vi "GetArmCount.vi"(8 "Error In":errorcluster, 11 "Keithley 7001 In":refnum<visa-resource-name>) -> (0 "Error Out":errorcluster, 1 "Infinite?":bool, 2 "Count?":u32, 3 "Keithley 7001 Out":refnum<visa-resource-name>)   [LabVIEW 2012, in "Keithley-7001.lvlib"]
uses:
  Keithley-7001.lvlib
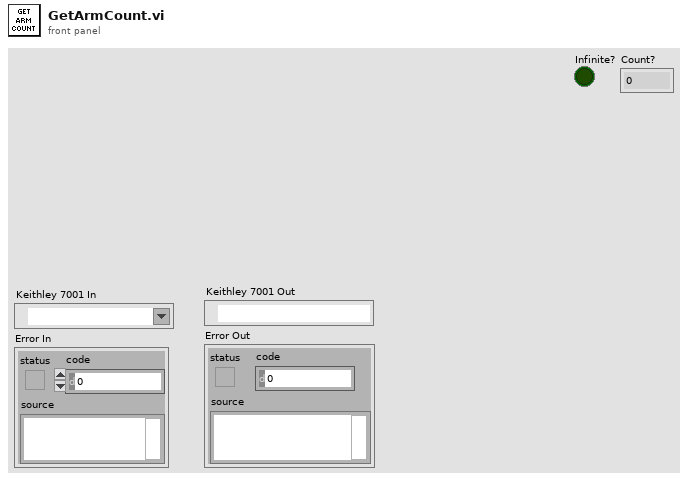
[diagram p1: front panel]
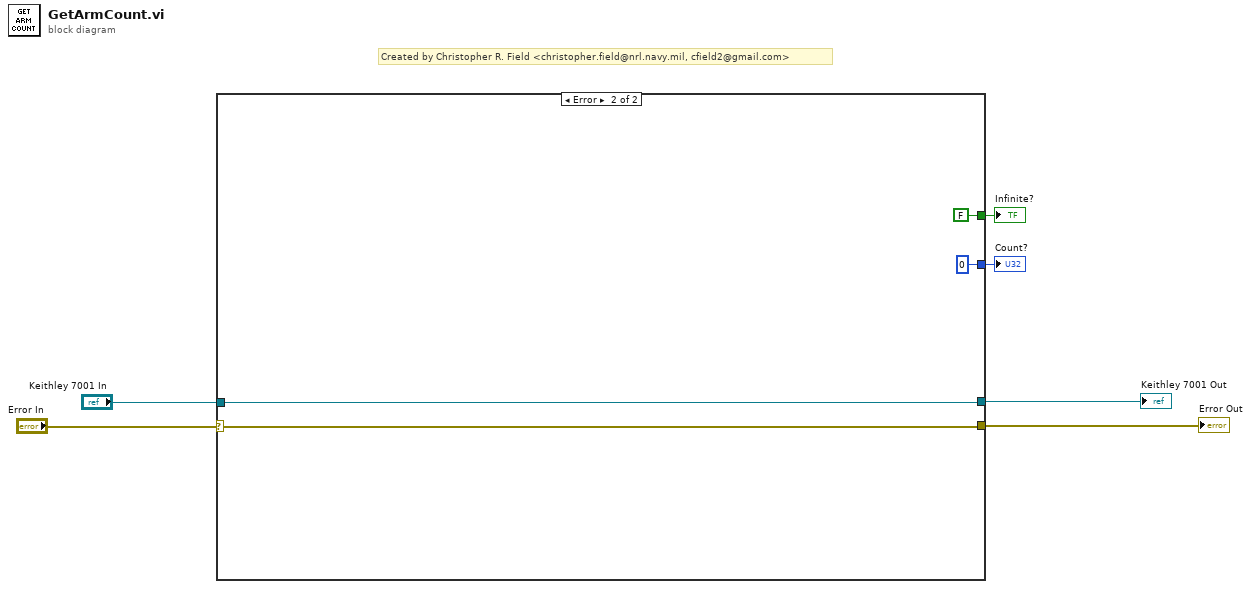
[diagram p0: block diagram]
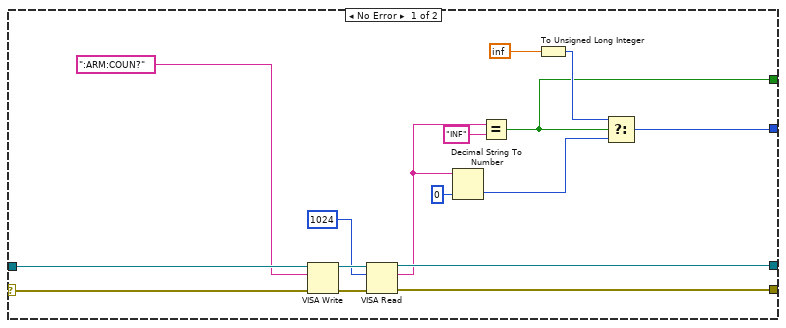
[diagram p2: hidden frame]
diagram:
  # "Created by Christopher R. Field <christopher.field@nrl.navy.mil, cfield2@gmail.com>"
  n1 = case shown="Error" "Error In" {
    selector: "Error In" -> [w15 w25]
    tunnel: "Keithley 7001 In" -> [w20 w26]
    tunnel: [w19 w26] -> w5
    tunnel: [w18 w25] -> w4
    tunnel: [w8 FALSE] -> w2
    tunnel: [w7 u32 0] -> w1
    frame No Error {
      n2 = VISA Write(VISA resource name=w20, write buffer=":ARM:COUN?", error in (no error)=w15) -> (VISA resource name out=w22:refnum<visa-resource-name>, error out=w21:errorcluster)  [unwired: 1 out]
      n3 = VISA Read(VISA resource name=w22, byte count=u32 1024, error in (no error)=w21) -> (VISA resource name out=w19:refnum<visa-resource-name>, read buffer=w13:string, error out=w18:errorcluster)  [unwired: 1 out]
      n4 = Decimal String To Number(string=w13, default (0L)=u32 0 ("default (0 I32)")) -> (number=w11:u32)  [unwired: 1 in, 1 out]
      n5 = Equal?(x=w13, y="INF") -> (x = y?=w8:bool)
      n6 = To Unsigned Long Integer(number=inf) -> (unsigned 32bit integer=w9:u32)
      n7 = Select(t=w9, s=w8, f=w11) -> (s? t:f=w7:u32)
    }
    frame Error {
    }
  }
  "Keithley 7001 Out" <- w5
  "Error Out" <- w4
  "Infinite?" <- w2
  "Count?" <- w1
